vi "Write Original.vi"(8 "error in (no error)":errorcluster, 10 "Original":bool, 11 "Task_Abstr in":refnum<class "Task_Abstr.lvclass">) -> (0 "error out":errorcluster, 3 "Task_Abstr out":refnum<class "Task_Abstr.lvclass">)   [LabVIEW 2025, in "Task_Abstr.lvlib" / "Task_Abstr.lvclass"]
uses:
  Task_Abstr.lvclass
  Task_Abstr.lvclass/Task_Abstr.ctl
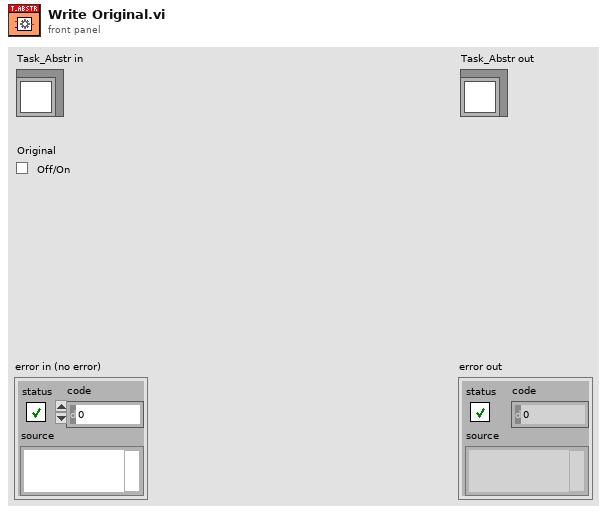
[diagram p1: front panel]
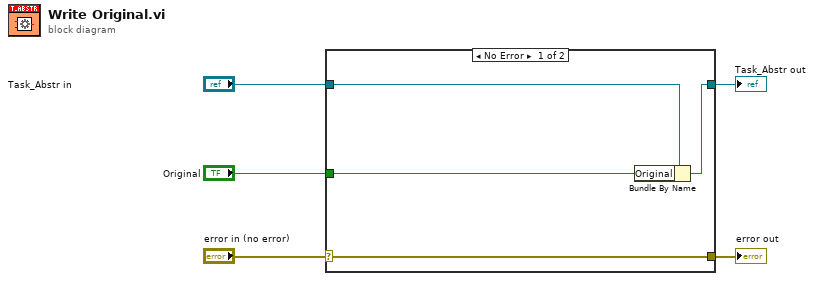
[diagram p0: block diagram]
diagram:
  n1 = case shown="No Error" "error in (no error)" {
    selector: "error in (no error)" -> [w9 w10]
    tunnel: [w9 w10] -> w4
    tunnel: [w7 w11] -> w2
    tunnel: "Task_Abstr in" -> [w8 w11]
    tunnel: "Original" -> [w6 _]
    frame No Error {
      n2 = Bundle By Name(cluster=w8, "Original"=w6) -> (w7:refnum<class "Task_Abstr.lvclass">)
    }
    frame Error {
    }
  }
  "error out" <- w4
  "Task_Abstr out" <- w2
